vi "ElectricalSorage.vi"(5 "Day of Year":u32, 6 "Unique Object Identifier":string, 7 "Day Time":u32, 8 "Error In":errorcluster, 10 "Energy flow IN":T6, 11 "DataFlowIN":T5) -> (0 "Error Out":errorcluster, 1 "El. Sorage Loading":cluster{"Load":bool, "Unload":bool}, 2 "Energy flow OUT":T6, 3 "DataFlowOUT":T5, 4 "Sorage Level":T2)   [LabVIEW 2017]
uses:
  classes/DataCollector.lvclass
  classes/DataHandler.lvclass
  classes/SimulationParameter.lvclass
panel:
  in  "Operating Parameter":T1
  out "Simulation Parameter":T3
  out "Control Parameter":T4
  out "List of Fieldelements":string[](array[string])
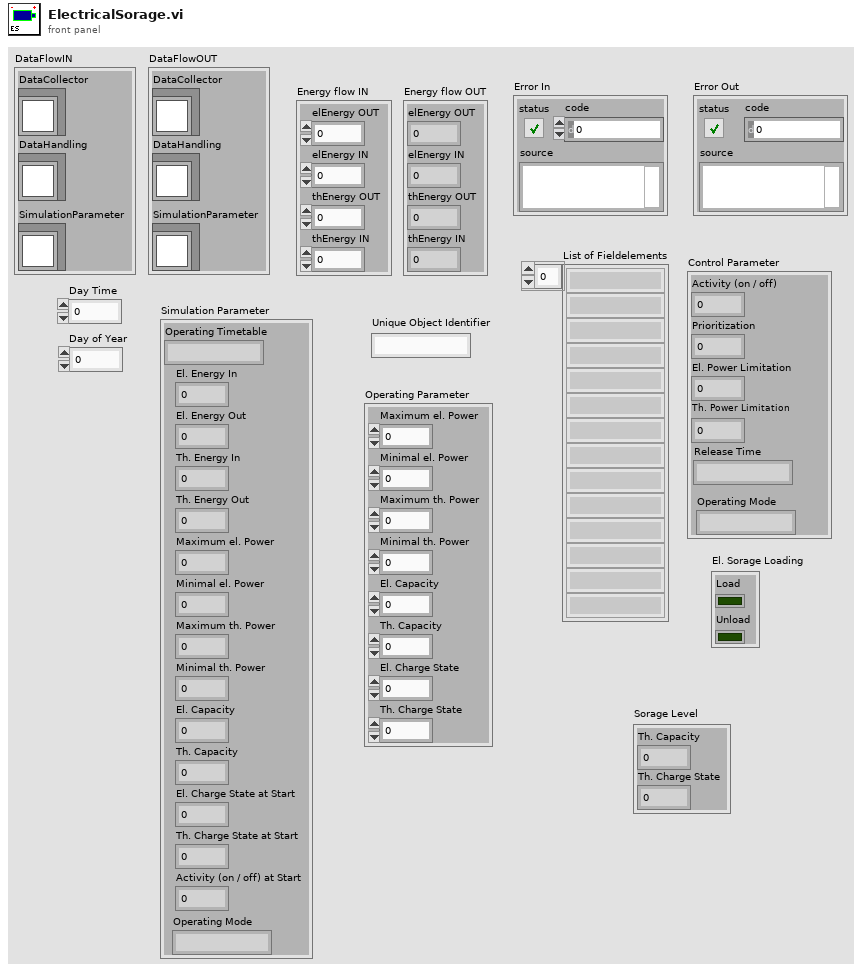
[diagram p1: front panel]
types:
  T1 = cluster{"Maximum el. Power":dbl, "Minimal el. Power":dbl, "Maximum th. Power":dbl, "Minimal th. Power":dbl, "El. Capacity":dbl, "Th. Capacity":dbl, "El. Charge State":dbl, "Th. Charge State":dbl}
  T2 = cluster{"Th. Capacity":dbl, "Th. Charge State":dbl}
  T3 = cluster{"Operating Timetable":string, "El. Energy In":dbl, "El. Energy Out":dbl, "Th. Energy In":dbl, "Th. Energy Out":dbl, "Maximum el. Power":dbl, "Minimal el. Power":dbl, "Maximum th. Power":dbl, "Minimal th. Power":dbl, "El. Capacity":dbl, "Th. Capacity":dbl, "El. Charge State at Start":dbl, "Th. Charge State at Start":dbl, "Activity (on / off) at Start":i64, "Operating Mode":string}
  T4 = cluster{"Activity (on / off)":i64, "Prioritization":i64, "El. Power Limitation":dbl, "Th. Power Limitation":dbl, "Release Time":string, "Operating Mode":string}
  T5 = cluster{"DataCollector":refnum<class "DataCollector.lvclass">, "DataHandling":refnum<class "DataHandler.lvclass">, "SimulationParameter":refnum<class "SimulationParameter.lvclass">}
  T6 = cluster{"elEnergy OUT":dbl, "elEnergy IN":dbl, "thEnergy OUT":dbl, "thEnergy IN":dbl}
  T7 = cluster{"El. Charge State":dbl, "Th. Charge State":dbl}
  T8 = cluster{"elEnergy OUT":dbl, "thEnergy OUT":dbl, "thEnergy IN":dbl, "thEnergy IN":dbl}
  T9 = cluster{"Day Time":u32, "Day of Year":u32, cluster{"elEnergy OUT":dbl, "thEnergy OUT":dbl, "thEnergy IN":dbl, "thEnergy IN":dbl}, "Operating Parameter":cluster{"Maximum el. Power":dbl, "Minimal el. Power":dbl, "Maximum th. Power":dbl, "Minimal th. Power":dbl, "El. Capacity":dbl, "Th. Capacity":dbl, "El. Charge State":dbl, "Th. Charge State":dbl}, "Control Parameter":cluster{"Activity (on / off)":i64, "Prioritization":i64, "El. Power Limitation":dbl, "Th. Power Limitation":dbl, "Release Time":string, "Operating Mode":string}}
  T10 = cluster{"thEnergy IN":dbl, "thEnergy IN":dbl, "elEnergy OUT":dbl, "thEnergy OUT":dbl}
  T11 = cluster{"Day Time":u32, "Day of Year":u32, cluster{"thEnergy IN":dbl, "thEnergy IN":dbl, "elEnergy OUT":dbl, "thEnergy OUT":dbl}, "Operating Parameter":cluster{"Maximum el. Power":dbl, "Minimal el. Power":dbl, "Maximum th. Power":dbl, "Minimal th. Power":dbl, "El. Capacity":dbl, "Th. Capacity":dbl, "El. Charge State":dbl, "Th. Charge State":dbl}, "Control Parameter":cluster{"Activity (on / off)":i64, "Prioritization":i64, "El. Power Limitation":dbl, "Th. Power Limitation":dbl, "Release Time":string, "Operating Mode":string}}
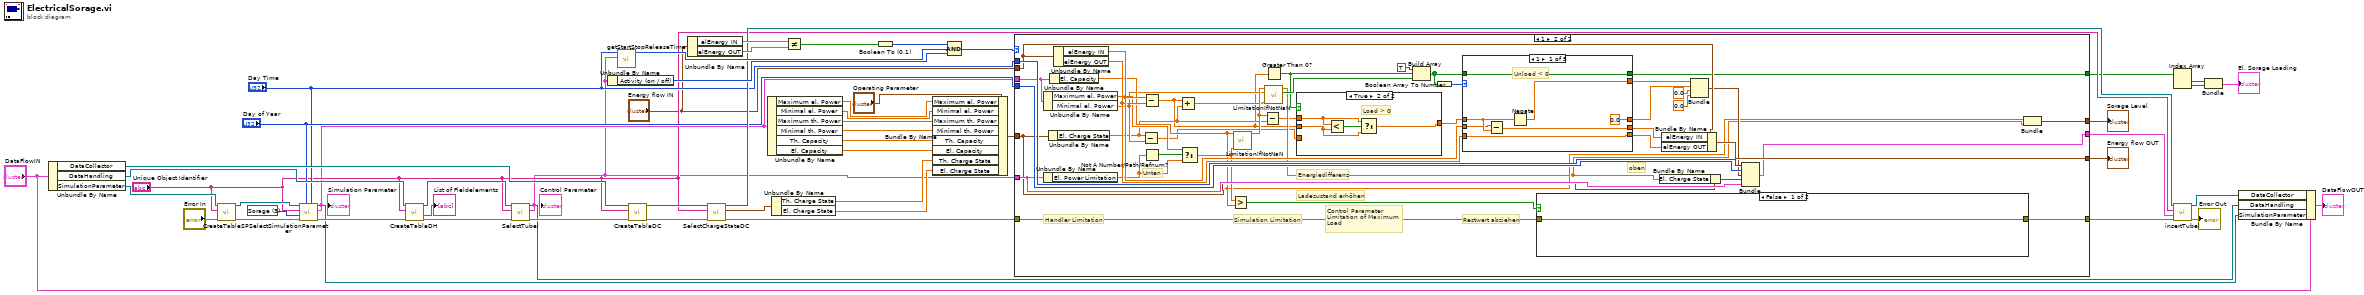
[diagram p0: block diagram]
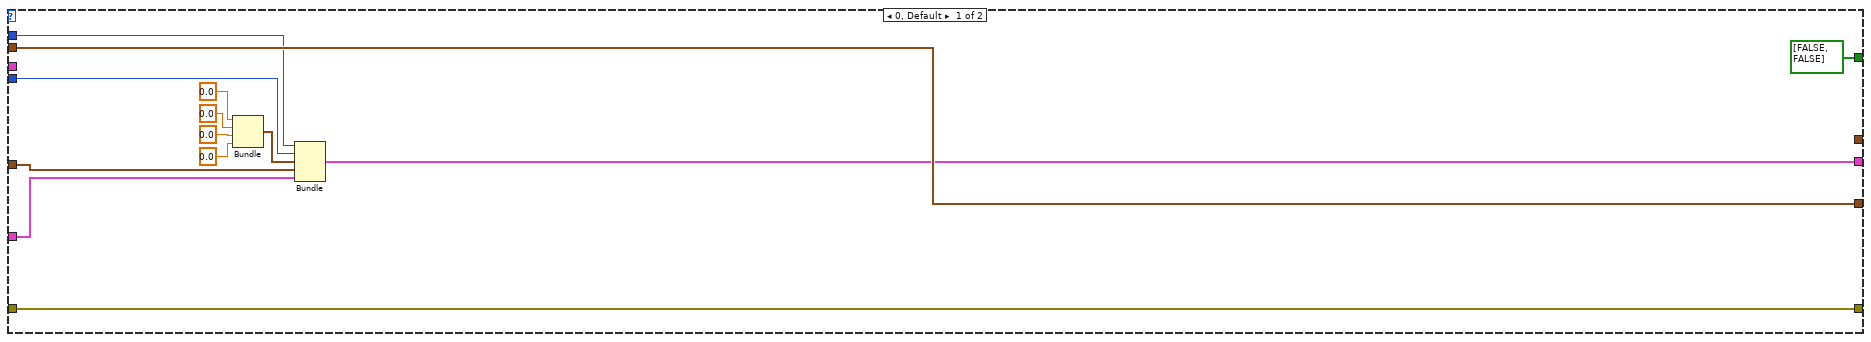
[diagram p2: hidden frame]
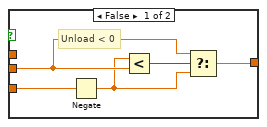
[diagram p3: hidden frame]
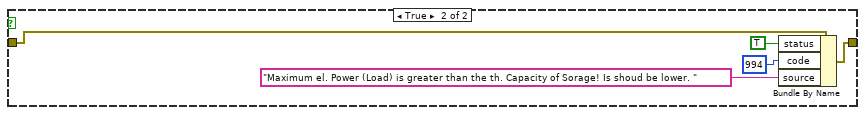
[diagram p4: hidden frame]
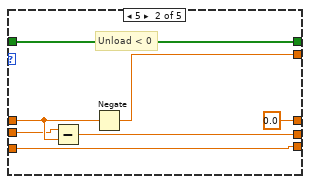
[diagram p5: hidden frame]
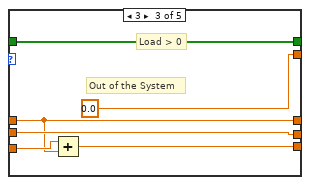
[diagram p6: hidden frame]
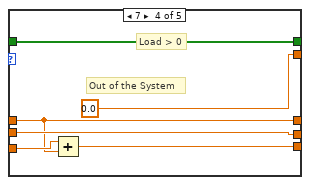
[diagram p7: hidden frame]
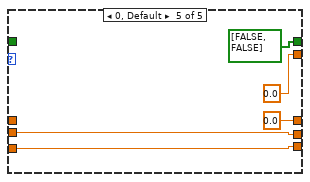
[diagram p8: hidden frame]
diagram:
  w19 = u16 3 items=["External Network", "Consumer", "Producer", "Sorage"] ("Type of Simulation")
  n1 = Unbundle By Name("DataFlowIN") -> ("DataCollector"=w54:refnum<class "DataCollector.lvclass">, "DataHandling"=w49:refnum<class "DataHandler.lvclass">, "SimulationParameter"=w44:refnum<class "SimulationParameter.lvclass">)
  n2 = call-dynamic "CreateTableSP.vi"("error in (no error)"="Error In", "Name of Table"="Unique Object Identifier", "SimulationParameter in"=w44) -> ("error out"=w47:errorcluster, "SimulationParameter out"=w46:refnum<class "SimulationParameter.lvclass">)  [unwired: 5 in, 2 out]
  n3 = call-dynamic "SelectSimulationParameter.vi"("Day of Year"="Day Time", "Day Time"="Day of Year", "error in (no error)"=w47, "Type of Simulation"=w19, "Unique Object Identifier"="Unique Object Identifier", "SimulationParameter in"=w46) -> ("error out"=w45:errorcluster, "Cluster"=w2:T3, "SimulationParameter out"=w43:refnum<class "SimulationParameter.lvclass">)  [unwired: 3 in]
  "Simulation Parameter" <- w2
  n4 = call-dynamic "CreateTableDH.vi"("error in (no error)"=w45, "Name of Table"="Unique Object Identifier", "DataHandler in"=w49) -> ("error out"=w52:errorcluster, "List of Fieldelements"=→"List of Fieldelements":string[], "DataHandler out"=w50:refnum<class "DataHandler.lvclass">)  [unwired: 5 in, 1 out]
  n5 = call-dynamic "SelectTubel.vi"("error in (no error)"=w52, "Unique Object Identifier"="Unique Object Identifier", "DataHandler in"=w50) -> ("error out"=w51:errorcluster, "Control Parameter"=w1:T4, "DataHandler out"=w48:refnum<class "DataHandler.lvclass">)  [unwired: 6 in]
  "Control Parameter" <- w1
  n6 = Unbundle By Name(w1) -> ("Activity (on / off)"=w38:i64)
  n7 = call "getStartStopReleaseTime.vi"("Control Parameter"=w1, "Day Time"="Day Time") -> ("Activity (on / off)"=w39:i64)  [unwired: 9 in]
  n8 = call "CreateTableDC.vi"("error in (no error)"=w51, "Name of Table"="Unique Object Identifier", "DataCollector in"=w54) -> ("error out"=w30:errorcluster, "DataCollector out"=w28:refnum<class "DataCollector.lvclass">)  [unwired: 7 in]
  n9 = Unbundle By Name("Energy flow IN") -> ("elEnergy IN"=w36:dbl, "elEnergy OUT"=w35:dbl)
  n10 = call-dynamic "SelectChargeStateDC.vi"("error in (no error)"=w30, "Unique Object Identifier"="Unique Object Identifier", "DataCollector in"=w28) -> ("error out"=w29:errorcluster, "Charge State"=w26:T7, "DataCollector out"=w27:refnum<class "DataCollector.lvclass">)  [unwired: 6 in]
  n11 = Unbundle By Name(w2) -> ("Maximum el. Power"=w23:dbl, "Minimal el. Power"=w22:dbl, "Maximum th. Power"=w33:dbl, "Minimal th. Power"=w32:dbl, "Th. Capacity"=w31:dbl, "El. Capacity"=w21:dbl)
  n12 = Unbundle By Name(w26) -> ("Th. Charge State"=w25:dbl, "El. Charge State"=w20:dbl)
  n13 = Not Equal?(x=w36, y=w35) -> (x != y?=w34:bool)
  n14 = Boolean To (0,1)(Boolean=w34) -> (0, 1=w40:i16)
  n15 = Bundle By Name(cluster="Operating Parameter", "Maximum el. Power"=w23, "Minimal el. Power"=w22, "Maximum th. Power"=w33, "Minimal th. Power"=w32, "Th. Capacity"=w31, "El. Capacity"=w21, "Th. Charge State"=w25, "El. Charge State"=w20) -> (w3:T1)
  n16 = Compound Arithmetic op=AND(w40, w39, w38) -> (w37:i64)
  n17 = case shown="1" w37 {
    tunnel: w29 -> [w66 w97]
    tunnel: [w66 w96] -> w42
    tunnel: "Day Time" -> [w59 w109]
    tunnel: "Day of Year" -> [w58 w108]
    tunnel: w3 -> [w61 w91]
    tunnel: "Energy flow IN" -> [w67 w107]
    tunnel: [w67 w105] -> w8
    tunnel: w2 -> [_ w106]
    tunnel: w1 -> [w56 w103]
    tunnel: [w57 w68] -> w41
    tunnel: [_ w89] -> w10
    tunnel: [bool[] [FALSE, FALSE] w84] -> w4
    frame 0, Default {
      n18 = Bundle("elEnergy OUT"=0.0, "thEnergy OUT"=0.0, "thEnergy IN"=0.0, "thEnergy IN"=0.0) -> (w60:T8)  [unwired: 1 in]
      n19 = Bundle("Day Time"=w59, "Day of Year"=w58, w60, "Operating Parameter"=w61, "Control Parameter"=w56) -> (w57:T9)  [unwired: 1 in]
    }
    frame 1 {
      # "Unten"
      # "oben"
      # "Energiedifferenz"
      # "Ladezustand erhöhen"
      # "Restwert abziehen"
      # "Control Parameter \nLimitation of Maximum \nLoad"
      # "Simulation Limitation"
      # "Handler Limitation"
      n20 = Unbundle By Name(w106) -> ("Maximum el. Power"=w93:dbl, "Minimal el. Power"=w80:dbl)
      n21 = Unbundle By Name(w103) -> ("El. Power Limitation"=w82:dbl)
      n22 = Unbundle By Name(w91) -> ("El. Charge State"=w79:dbl)
      n23 = Unbundle By Name(w106) -> ("El. Capacity"=w90:dbl)
      n24 = Unbundle By Name(w107) -> ("elEnergy IN"=w102:dbl, "elEnergy OUT"=w101:dbl)
      n25 = Subtract(x=w79, y=w80) -> (x-y=w70:dbl)
      n26 = Subtract(x=w102, y=w101) -> (x-y=w73:dbl)
      n27 = Not A Number/Path/Refnum?(number/path/refnum=w82) -> (NaN/Path/Refnum?=w94:bool)
      n28 = Add(x=w73, y=w79) -> (x+y=w75:dbl)
      n29 = Select(t=w93, s=w94, f=w82) -> (s? t:f=w92:dbl)
      n30 = Greater?(x=w92, y=w90) -> (0:w95:bool)
      n31 = call "LimitationIfNotNaN.vi"("x"=w92, "Maximum Power"=w90) -> ("Power Out"=w81:dbl)  [unwired: 8 in, 1 out]
      n32 = Subtract(x=w81, y=w79) -> (x-y=w74:dbl)
      n33 = Greater Than 0?(x=w73) -> (x > 0?=w77:bool)
      n34 = call "LimitationIfNotNaN.vi"("x"=w75, "Minimal Power"=w80, "Maximum Power"=w81) -> ("In Range?"=w83:bool, "Power Out"=w76:dbl)  [unwired: 7 in]
      n35 = case shown="True" w77 {
        tunnel: w73 -> [w111 w116]
        tunnel: w74 -> [_ w115]
        tunnel: [w113 w118] -> w71
        tunnel: w70 -> [w112 _]
        frame False {
          # "Unload < 0"
          n36 = Negate(x=w112) -> (-x=w110:dbl)
          n37 = Less?(x=w110, y=w111) -> (x < y?=w114:bool)
          n38 = Select(t=w111, s=w114, f=w110) -> (s? t:f=w113:dbl)
        }
        frame True {
          # "Load > 0"
          n39 = Less?(x=w115, y=w116) -> (x < y?=w117:bool)
          n40 = Select(t=w115, s=w117, f=w116) -> (s? t:f=w118:dbl)
        }
      }
      n41 = Build Array(TRUE ("element"), w77, w83) -> (w85:bool[])
      n42 = Boolean Array To Number(Boolean array=w85) -> (number=w98:u32)
      n43 = case shown="1" w98 {
        tunnel: w102 -> [w126 w133 w140 w146 w152]
        tunnel: w71 -> [w128 w135 w139 w145 _]
        tunnel: w101 -> [w125 w132 w141 w147 w151]
        tunnel: [w127 w134 w140 w146 w152] -> w100
        tunnel: [w125 w132 w142 w148 w151] -> w99
        tunnel: [w130 w137 0.0 ("thEnergy IN") 0.0 ("thEnergy IN") 0.0 ("thEnergy IN")] -> w88
        tunnel: [w129 w136 w143 w149 bool[] [FALSE, FALSE]] -> w84
        tunnel: w85 -> [w129 w136 w143 w149 _]
        tunnel: [0.0 ("thEnergy IN") 0.0 ("thEnergy IN") w139 w145 0.0 ("thEnergy IN")] -> w78
        frame 1 {
          # "Unload < 0"
          n44 = Subtract(x=w126, y=w128) -> (x-y=w127:dbl)
          n45 = Negate(x=w128) -> (-x=w130:dbl)
        }
        frame 5 {
          # "Unload < 0"
          n46 = Subtract(x=w133, y=w135) -> (x-y=w134:dbl)
          n47 = Negate(x=w135) -> (-x=w137:dbl)
        }
        frame 3 {
          # "Out of the System"
          # "Load > 0"
          n48 = Add(x=w141, y=w139) -> (x+y=w142:dbl)
        }
        frame 7 {
          # "Out of the System"
          # "Load > 0"
          n49 = Add(x=w147, y=w145) -> (x+y=w148:dbl)
        }
        frame 0, Default {
        }
      }
      n50 = case shown="False" w95 {
        tunnel: w97 -> [w119 w124]
        tunnel: [w119 w123] -> w96
        frame False {
        }
        frame True {
          n51 = Bundle By Name(cluster=w124, "status"=TRUE, "code"=994, "source"="Maximum el. Power (Load) is greater than the th. Capacity of Sorage! Is shoud be lower. ") -> (w123:errorcluster)
        }
      }
      n52 = Bundle By Name(cluster=w91, "El. Charge State"=w76) -> (w69:T1)
      n53 = Bundle By Name(cluster=w107, "elEnergy IN"=w100, "elEnergy OUT"=w99) -> (w105:T6)
      n54 = Bundle("thEnergy IN"=w88, "thEnergy IN"=w78, "elEnergy OUT"=0.0, "thEnergy OUT"=0.0) -> (w104:T10)  [unwired: 1 in]
      n55 = Bundle("Day Time"=w109, "Day of Year"=w108, w104, "Operating Parameter"=w69, "Control Parameter"=w103) -> (w68:T11)  [unwired: 1 in]
      n56 = Bundle("El. Capacity"=w90, "Power Out"=w76) -> (w89:cluster{"El. Capacity":dbl, "Power Out":dbl})  [unwired: 1 in]
    }
  }
  "Energy flow OUT" <- w8
  "Sorage Level" <- w10
  n57 = Index Array(array=w4) -> (element #1=w6:bool, element #2=w7:bool)  [unwired: 2 in]
  n58 = call-dynamic "insertTubel.vi"("error in (no error)"=w42, "Data Cluster"=w41, "Name of Table"="Unique Object Identifier", "DataCollector in"=w27) -> ("error out"=→"Error Out":errorcluster, "DataCollector out"=w53:refnum<class "DataCollector.lvclass">)  [unwired: 6 in]
  n59 = Bundle("In Range?"=w6, "In Range?"=w7) -> (→"El. Sorage Loading":cluster{"In Range?":bool, "In Range?":bool})  [unwired: 1 in]
  n60 = Bundle By Name(cluster="DataFlowIN", "DataCollector"=w53, "DataHandling"=w48, "SimulationParameter"=w43) -> (→"DataFlowOUT":T5)
